vi "Get_Win_Names.vi"(3 "error in":errorcluster) -> (7 "Win_Names":string[](array[string]), 10 "error out":errorcluster)   [LabVIEW 2025]
uses:
  user32.dll
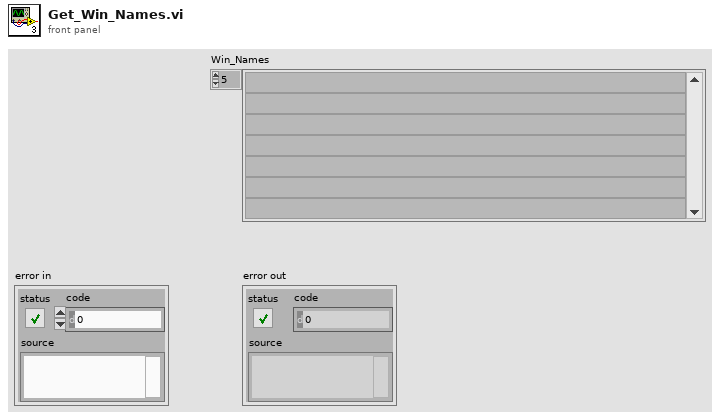
[diagram p1: front panel]
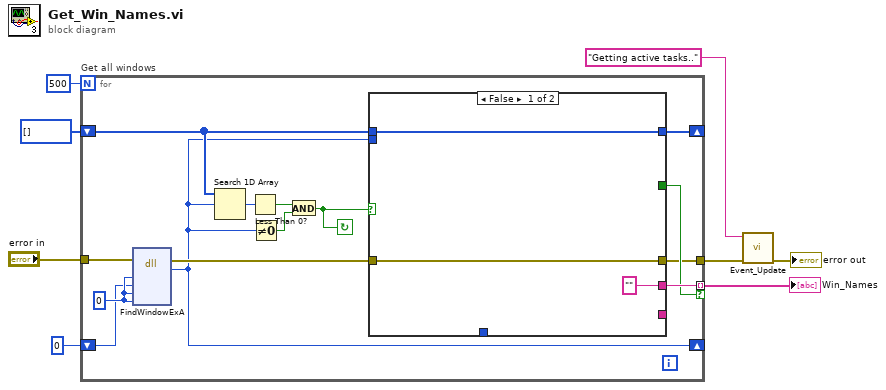
[diagram p0: block diagram]
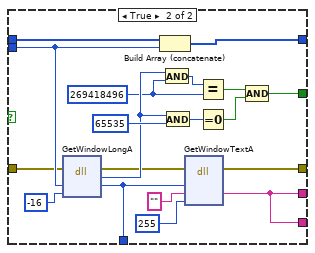
[diagram p2: hidden frame]
diagram:
  n1 = for "Get all windows" {
    N: 500 -> [_]
    shift-right: [w10] -> _
    shift-left: 0 ("hWnd") -> [w21]
    shift-right: [w20] -> _
    shift-left: i32[] [] -> [w19]
    tunnel: [w14] -> w4 mode=indexing if=w13
    tunnel: [w12] -> w3
    tunnel: "error in" -> [w11]
    stop <- w9 continue-if-true
    w22 = 0 ("classname")
    n2 = dll-call lib="user32.dll" fn="FindWindowExA" ("kernel32:FindWindowEx")(error in=w11, "hWnd parent"=w22, "hWnd previous"=w21, "classname"=w22, "window name"=w22) -> (error out=w15:errorcluster, "hWnd"=w10:i32)  [unwired: 6 in, 1 out]
    n3 = Search 1D Array(1D array=w19, element=w10) -> (index of element=w18:i32)  [unwired: 1 in]
    n4 = Less Than 0?(x=w18) -> (x < 0?=w17:bool)
    n5 = Not Equal To 0?(x=w10) -> (x != 0?=w16:bool)
    n6 = And(x=w17, y=w16) -> (x .and. y?=w9:bool)
    n7 = case shown="False" w9 {
      tunnel: w10 -> [_ w32]
      tunnel: w19 -> [w25 w44]
      tunnel: [w25 w43] -> w20
      tunnel: w15 -> [w23 w31]
      tunnel: ["" ("hWnd") w26] -> w14
      tunnel: [_ w29] -> w13
      tunnel: [w23 w28] -> w12
      tunnel: [_ w27] -> _
      tunnel: [_ w26] -> _
      frame False {
      }
      frame True {
        w33 = 269418496 ("y")
        n8 = dll-call lib="user32.dll" fn="GetWindowLongA" ("kernel32:FindWindowEx")(error in=w31, "hWnd"=w32, "index"=-16) -> (error out=w30:errorcluster, "hWnd"=w35:i32, "hWnd"=w27:i32)  [unwired: 3 in, 1 out]
        n9 = Build Array (concatenate)(w44, w32) -> (w43:i32[])
        n10 = And(x=w35, y=w33) -> (x .and. y?=w41:i32)
        n11 = And(x=w35, y=65535) -> (x .and. y?=w39:i32)
        n12 = dll-call lib="user32.dll" fn="GetWindowTextA" ("kernel32:FindWindowEx")(error in=w30, "hWnd"=w27, "hWnd"="", "size"=255) -> (error out=w28:errorcluster, "hWnd"=w26:string)  [unwired: 5 in, 1 out]
        n13 = Equal?(x=w41, y=w33) -> (x = y?=w36:bool)
        n14 = Equal To 0?(x=w39) -> (x = 0?=w34:bool)
        n15 = Compound Arithmetic op=AND(w36, w34) -> (w29:bool)
      }
    }
  }
  "Win_Names" <- w4
  n16 = call "Event_Update.vi"("Error In"=w3, "Event"="Getting active tasks..") -> ("Error Out"=→"error out":errorcluster)  [unwired: 9 in]
